vi "BigIntDevidedByU32.vi"(2 "b (<1e9)":u64, 3 "a":cluster{"Boolean":bool, "Array":u64[]}) -> (0 "a % b":cluster{"Boolean":bool, "Array":u64[]}, 1 "a / b":cluster{"Boolean":bool, "Array":u64[]})   [LabVIEW 2023]
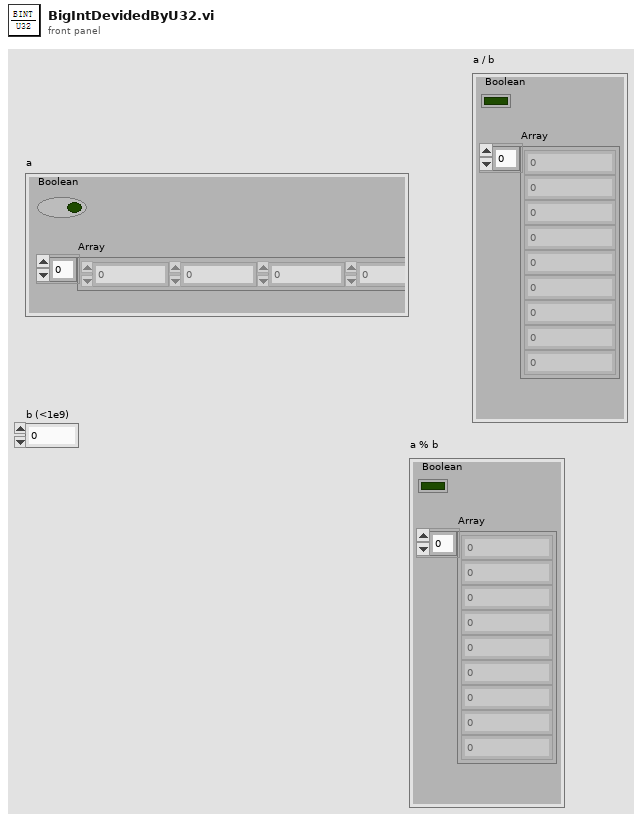
[diagram p1: front panel]
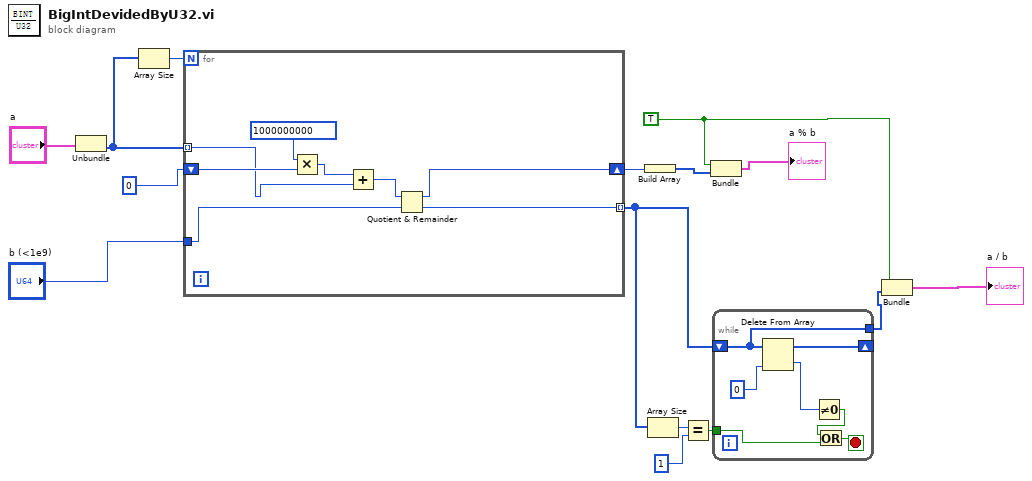
[diagram p0: block diagram]
diagram:
  w10 = TRUE
  n1 = Unbundle("a") -> ("Array"=w13:u64[])  [unwired: 1 out]
  n2 = Array Size(array=w13) -> (size(s)=w14:i32)
  n3 = for {
    N: w14 -> [_]
    tunnel: w13 -> [w18] mode=indexing
    tunnel: "b (<1e9)" -> [w23]
    tunnel: [w22] -> w4 mode=indexing
    shift-right: [w21] -> w11
    shift-left: u64 0 -> [w20]
    n4 = Multiply(x=u64 1000000000, y=w20) -> (x*y=w17:u64)
    n5 = Add(x=w17, y=w18) -> (x+y=w16:u64)
    n6 = Quotient & Remainder(x=w16, y=w23) -> (x-y*floor(x/y)=w21:u64, floor(x/y)=w22:u64)
  }
  n7 = Build Array(w11) -> (w9:u64[])
  n8 = Array Size(array=w4) -> (size(s)=w3:i32)
  n9 = Equal?(x=w3, y=1) -> (x = y?=w1:bool)
  n10 = Bundle(w10, w9) -> (→"a % b":cluster{bool, u64[]})  [unwired: 1 in]
  n11 = while {
    shift-right: [w30] -> _
    shift-left: w4 -> [w29]
    tunnel: [w29] -> w5
    tunnel: w1 -> [w24]
    stop <- w25 stop-if-true
    n12 = Delete From Array(array=w29, index=0) -> (deleted portion=w27:u64, array with subset deleted=w30:u64[])  [unwired: 1 in]
    n13 = Not Equal To 0?(x=w27) -> (x != 0?=w26:bool)
    n14 = Or(x=w26, y=w24) -> (x .or. y?=w25:bool)
  }
  n15 = Bundle(w10, w5) -> (→"a / b":cluster{bool, u64[]})  [unwired: 1 in]
